vi "Get Class Methods.vi"(9 "LVClassLibrary Refnum":refnum<vi>) -> (1 "DataMembers":string[](array[string]), 2 "DynamicMembers":string[](array[string]), 3 "StaticMembers":string[](array[string]))   [LabVIEW 2020]
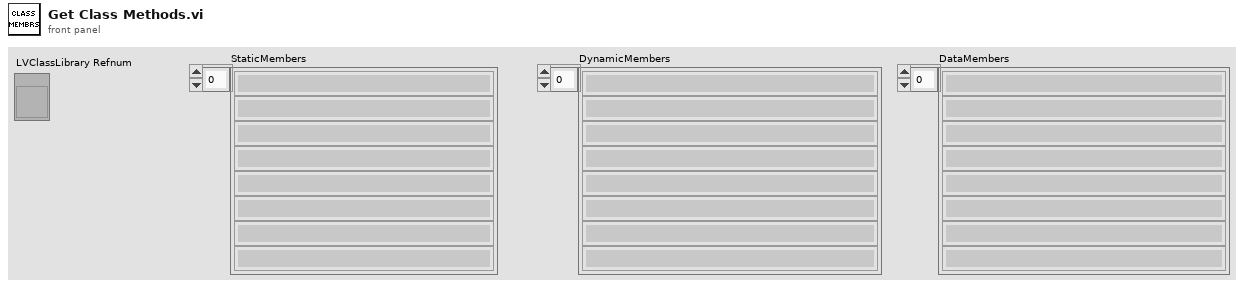
[diagram p1: front panel]
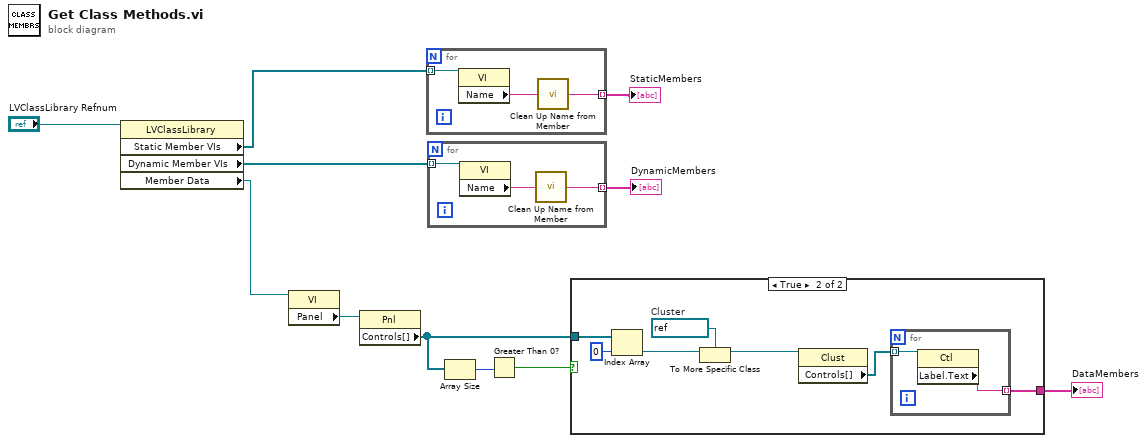
[diagram p0: block diagram]
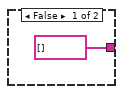
[diagram p2: hidden frame]
diagram:
  n1 = property class="LVClassLibrary"(reference="LVClassLibrary Refnum") -> ("Static Member VIs"=w10:refnum<vi>[], "Dynamic Member VIs"=w8:refnum<vi>[], "Member Data"=w7:refnum<vi>)  [unwired: 1 in, 2 out]
  n2 = property class="VI"(reference=w7) -> ("Panel"=w6:refnum<vi>)  [unwired: 1 in, 2 out]
  n3 = property class="Pnl"(reference=w6) -> ("Controls[]"=w3:refnum<vi>[])  [unwired: 1 in, 2 out]
  n4 = for {
    tunnel: w10 -> [w14] mode=indexing
    tunnel: [w12] -> w9 mode=indexing
    n5 = property class="VI"(reference=w14) -> ("Name"=w13:string)  [unwired: 1 in, 2 out]
    n6 = call "Clean Up Name from Member.vi"("Name Input"=w13) -> ("Clean Name Output"=w12:string)
  }
  "StaticMembers" <- w9
  n7 = for {
    tunnel: w8 -> [w17] mode=indexing
    tunnel: [w15] -> w1 mode=indexing
    n8 = property class="VI"(reference=w17) -> ("Name"=w16:string)  [unwired: 1 in, 2 out]
    n9 = call "Clean Up Name from Member.vi"("Name Input"=w16) -> ("Clean Name Output"=w15:string)
  }
  "DynamicMembers" <- w1
  n10 = Array Size(array=w3) -> (size(s)=w5:i32)
  n11 = Greater Than 0?(x=w5) -> (x > 0?=w4:bool)
  n12 = case shown="True" w4 {
    tunnel: w3 -> [_ w20]
    tunnel: [string[] [] w19] -> w2
    frame False {
    }
    frame True {
      w24 = refnum<vi> refnum  # Cluster
      n13 = Index Array(array=w20, index=0) -> (element=w23:refnum<vi>)
      n14 = To More Specific Class(target class=w24, reference=w23) -> (specific class reference=w22:refnum<vi>)  [unwired: 1 in, 1 out]
      n15 = property class="Clust"(reference=w22) -> ("Controls[]"=w21:refnum<vi>[])  [unwired: 1 in, 2 out]
      n16 = for {
        tunnel: w21 -> [w27] mode=indexing
        tunnel: [w26] -> w19 mode=indexing
        n17 = property class="Ctl"(reference=w27) -> ("Label.Text"=w26:string)  [unwired: 1 in, 2 out]
      }
    }
  }
  "DataMembers" <- w2
